vi "Dispose of Pointer.vi"(11 "Pointer":u32) -> ()   [LabVIEW 2021]
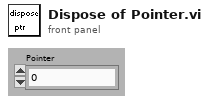
[diagram p1: front panel]
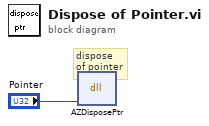
[diagram p0: block diagram]
diagram:
  # "dispose\nof pointer"
  n1 = dll-call lib="LabVIEW" fn="AZDisposePtr"("UPtr"="Pointer") -> ()  [unwired: 5 in, 2 out]
